vi "Init4503.vi"(0 "4503 in":refnum<class "4503.lvclass">, 1 "FetchDataRefs":refnum<vi>[](array[refnum]), 2 "InvertCWCCW":bool, 3 "Setting ref":refnum<vi>, 5 "TorqueSensor":T1={"Interface"="", "Read Unit"=enum."Kg.cm", "Encoder"=0, "Torque Filter"=0, "Max Torque"=2.0, "Max Power"=50.0, "Max Speed"=50.0, "Scale Factor CW"=2.0, "Scale Factor CCW"=2.0, "Scale Factor Zero"=2.0} {"Scale Factor Zero" format="%#.6f"; "Scale Factor CCW" format="%#.6f"; "Scale Factor CW" format="%#.6f"; "Torque Filter" items=["OFF", "10Hz", "25Hz", "50Hz", "3Hz", "2Hz", "1Hz"]; "Encoder" items=["60-ppr"=60, "600-ppr"=600, "6000-ppr"=6000, "8192-ppr"=8192, "20-ppr"=20, "30-ppr"=30, "1-ppr"=1, "2-ppr"=2, "6-ppr"=6]}, 9 "ref Dy Value":refnum<vi>, 11 "error in (no error)":errorcluster, 12 "CWCCW ref":refnum<vi>, 13 "Role":enum16{"Drive", "Load"}(ring)) -> (4 "4503 out":refnum<class "4503.lvclass">, 15 "error out":errorcluster)   [LabVIEW 2024, in "4503 Actor.lvlib" / "4503.lvclass"]
uses:
  4503.lvclass
  MFActor/SystemSettings.ctl
  4503.lvclass/4503.ctl
panel:
  out "AutoFetchData":refnum<vi>
  out "SampleRate":refnum<vi>
  out "ManualFetchData":refnum<vi>
  out "MASampleNum":refnum<vi>
  in  "SampleRate":u32=1 caption="Sec." min=1
  in  "AutoFetchData":bool
  in  "ManualFetchData":bool
  in  "MASampleNum":u32=1 caption="平均樣本數" min=1
  in  "Dy Value":T2 caption="Resule Value" {"AngleValue" format="%.2f"; "Wout" format="%.2f"; "Torque Value" format="%.2f"}
  in  "StopSignal":refnum<user-event>
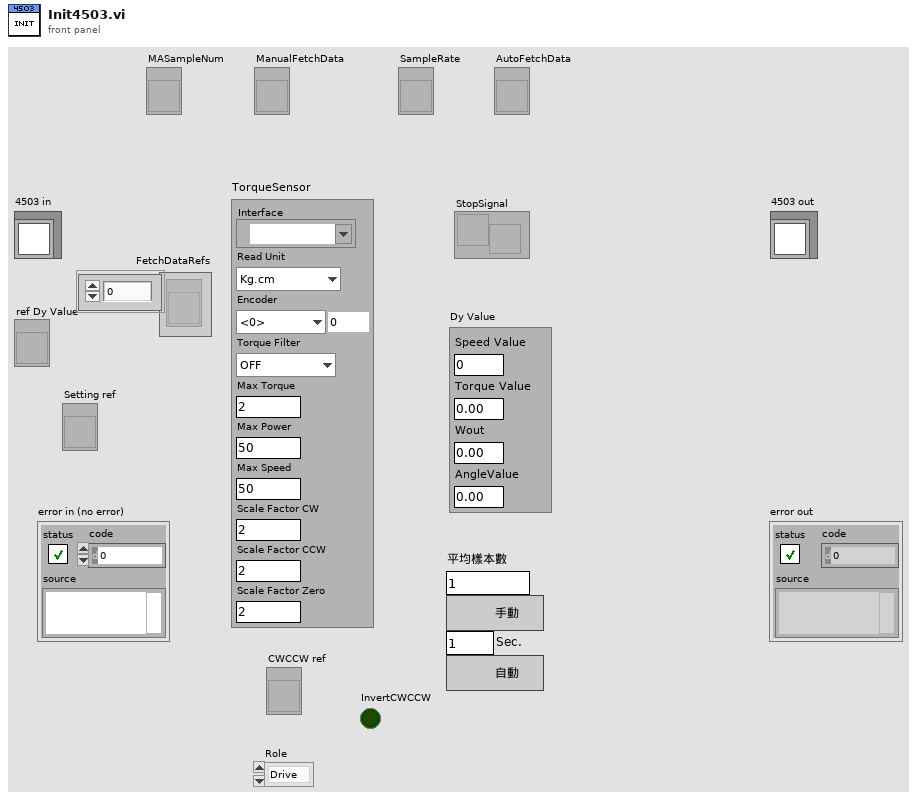
[diagram p1: front panel]
types:
  T1 = cluster{"Interface":refnum<visa-resource-name>, "Read Unit":enum16{"oz.in", "oz.ft", "lb.in", "lb.ft", "g.cm", "Kg.cm", "mN.m", "cN.m", "N.m"}, "Encoder":u16, "Torque Filter":u16, "Max Torque":dbl, "Max Power":dbl, "Max Speed":dbl, "Scale Factor CW":dbl, "Scale Factor CCW":dbl, "Scale Factor Zero":dbl}
  T2 = cluster{"Speed Value":dbl, "Torque Value":dbl, "Wout":dbl, "AngleValue":dbl}
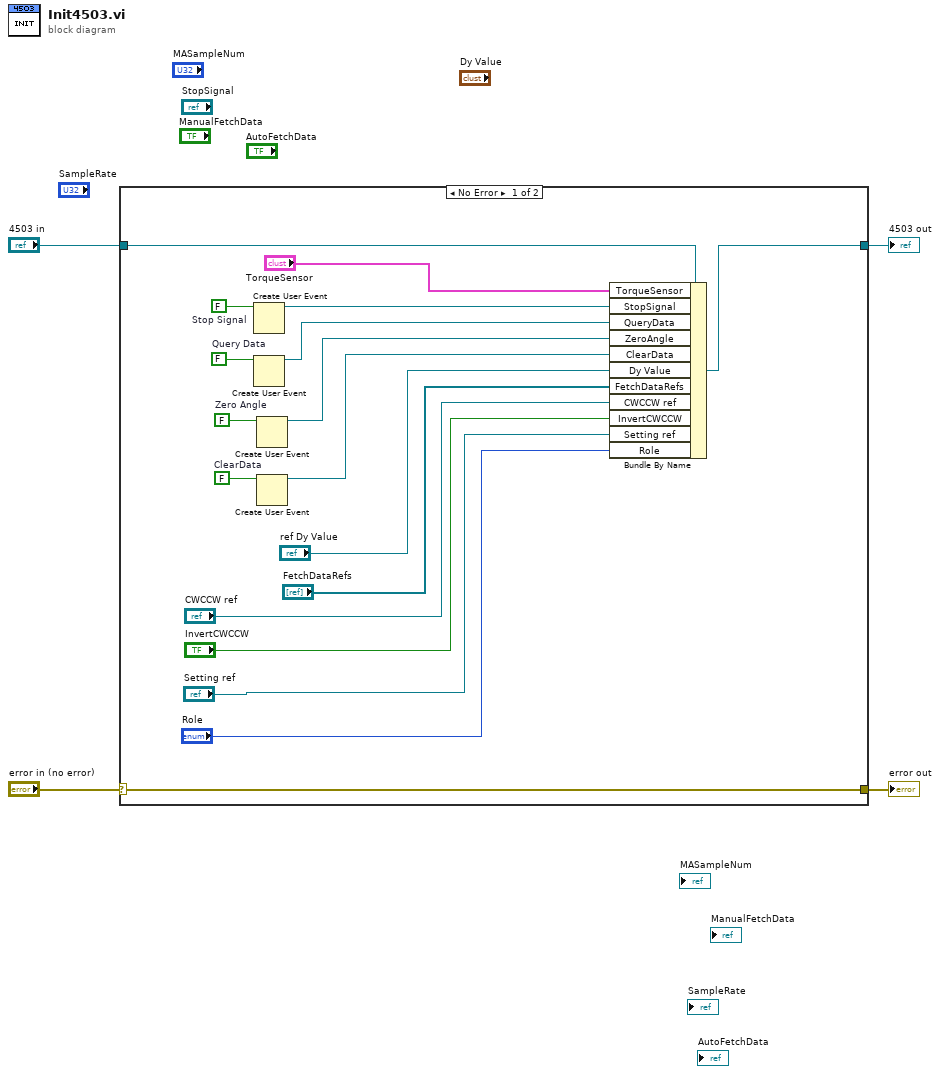
[diagram p0: block diagram]
diagram:
  n1 = case shown="No Error" "error in (no error)" {
    selector: "error in (no error)" -> [w22 w24]
    tunnel: [w22 w24] -> w3
    tunnel: [w16 w23] -> w1
    tunnel: "4503 in" -> [w17 w23]
    frame No Error {
      w6 = FALSE  # ClearData
      w8 = FALSE  # Zero Angle
      w10 = FALSE  # Query Data
      w20 = FALSE  # Stop Signal
      n2 = Create User Event(user event datatype=w20) -> (user event=w19:refnum<user-event>)  [unwired: 1 in, 1 out]
      n3 = Create User Event(user event datatype=w10) -> (user event=w9:refnum<user-event>)  [unwired: 1 in, 1 out]
      n4 = Create User Event(user event datatype=w8) -> (user event=w7:refnum<user-event>)  [unwired: 1 in, 1 out]
      n5 = Create User Event(user event datatype=w6) -> (user event=w5:refnum<user-event>)  [unwired: 1 in, 1 out]
      n6 = Bundle By Name(cluster=w17, "TorqueSensor"="TorqueSensor", "StopSignal"=w19, "QueryData"=w9, "ZeroAngle"=w7, "ClearData"=w5, "Dy Value"="ref Dy Value", "FetchDataRefs"="FetchDataRefs", "CWCCW ref"="CWCCW ref", "InvertCWCCW"="InvertCWCCW", "Setting ref"="Setting ref", "Role"="Role") -> (w16:refnum<class "4503.lvclass">)
    }
    frame Error {
    }
  }
  "error out" <- w3
  "4503 out" <- w1
